vi "CANOpen_NMT_Write HW Outputs.vi"(8 "error in":errorcluster, 9 "Node Ids":T1, 10 "Hardware Output FIFO":refnum<k33>, 11 "Channel Pairs":T2 {"Chan Refs"."Data Reference" format="%.0x"}) -> (0 "error out":errorcluster, 2 "Write Occured":bool, 3 "Channel Pairs":T2 {"Chan Refs"."Data Reference" format="%.0x"})   [LabVIEW 2021, in "CANOpen Addon Engine.lvlib"]
uses:
  CANOpen Addon Engine.lvlib
  CanOpen_NMT_HWOut_ChannelPairs.ctl
  <vilib>/NI VeriStand/Custom Device API/Block Data Reference.ctl
  <vilib>/NI VeriStand/Custom Device API/Data Reference.ctl
  CanOpen_Main Node Ids.ctl
  <vilib>/NI VeriStand/Custom Device API/Global Data Refs.vi
  <vilib>/NI VeriStand/Custom Device API/Custom Device API.lvlib
  Debug/SubVIs/Global debug.vi
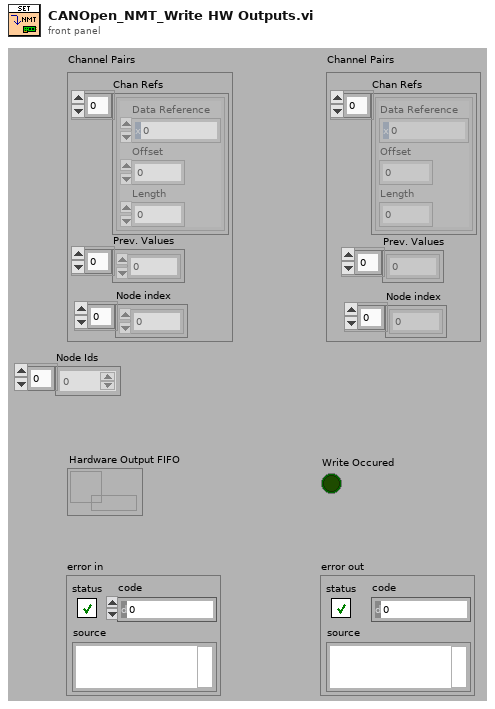
[diagram p1: front panel]
types:
  T1 = typedef "CANOpen Addon Engine.lvlib/CanOpen_Main Node Ids.ctl" = u8[]
  T2 = typedef "CANOpen Addon Engine.lvlib/CanOpen_NMT_HWOut_ChannelPairs.ctl" = cluster{"Chan Refs":T3[], "Prev. Values":dbl[], "Node index":dbl[]}
  T3 = typedef "Custom Device API.lvlib/Block Data Reference.ctl" = cluster{"Data Reference":T4, "Offset":u64, "Length":u64}
  T4 = typedef "Custom Device API.lvlib/Data Reference.ctl" = i32
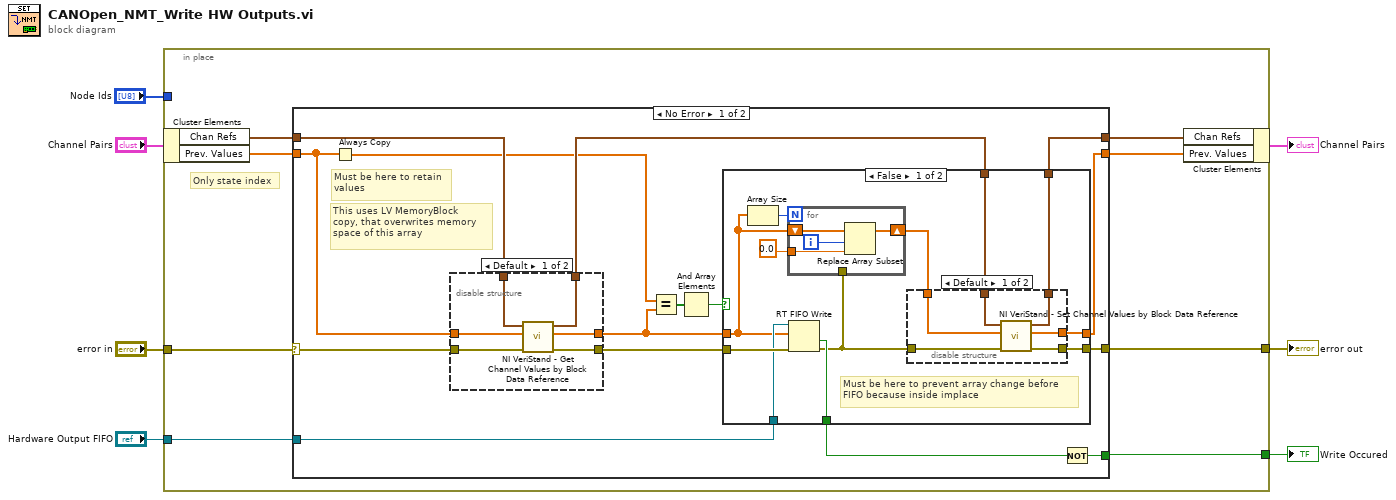
[diagram p0: block diagram]
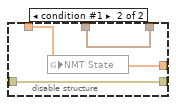
[diagram p2: hidden frame]
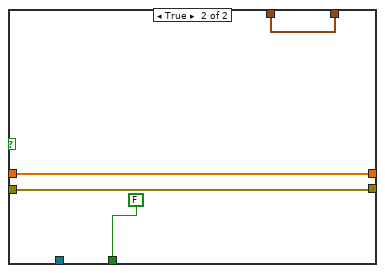
[diagram p3: hidden frame]
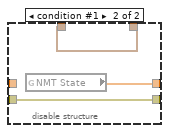
[diagram p4: hidden frame]
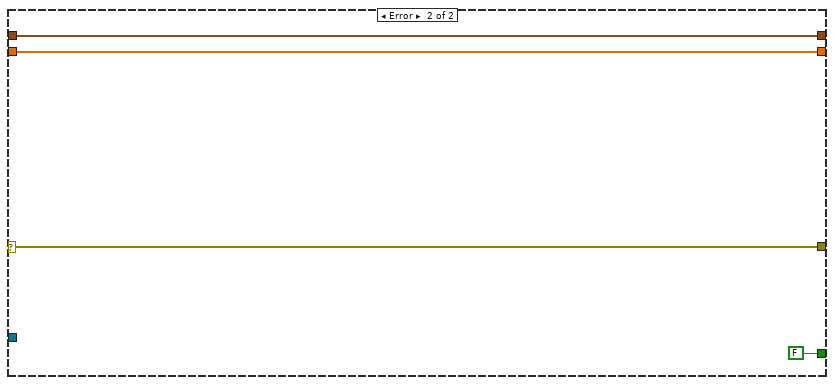
[diagram p5: hidden frame]
diagram:
  n1 = in-place {
    in-place-border: [w15] -> w7
    in-place-border: [w14] -> w6
    in-place-border: "error in" -> [w11]
    in-place-border: "Hardware Output FIFO" -> [w8]
    in-place-border: "Node Ids" -> [_]
    # "Only state index"
    n2 = in-place-cluster #1("Channel Pairs") -> ("Chan Refs"=w13:T3[], "Prev. Values"=w10:dbl[])
    n3 = case shown="No Error" w11 {
      selector: w11 -> [w27 w72]
      tunnel: [w28 w72] -> w15
      tunnel: [w19 w69] -> w9
      tunnel: [w29 FALSE ("C Read Occured?")] -> w14
      tunnel: w13 -> [w25 w70]
      tunnel: [w20 w70] -> w12
      tunnel: w10 -> [w16 w69]
      tunnel: w8 -> [w24 _]
      frame No Error {
        # "This uses LV MemoryBlock\ncopy, that overwrites memory\nspace of this array"
        # "Must be here to retain\nvalues"
        n4 = Always Copy(1:w16) -> (0:w17:dbl[])
        n5 = disable-structure shown="Default" {
          disable-tunnel: w27 -> [w65 w68]
          disable-tunnel: [w61 w68] -> w26
          disable-tunnel: w25 -> [w64 w67]
          disable-tunnel: [w63 w67] -> w21
          disable-tunnel: w16 -> [w62 _]
          disable-tunnel: [w60 w66] -> w18
          frame condition #0 (active) {
            n6 = call <vilib>:"NI VeriStand - Get Channel Values by Block Data Reference.vi"("error in (no error)"=w65, "Values Array in"=w62, "Block Data Ref"=w64) -> ("error out"=w61:errorcluster, "Values Array out"=w60:dbl[], "Block Data Ref dup"=w63:T3[])  [unwired: 6 in]
          }
          frame condition #1 {
            n7 = global read "Global debug.vi" "NMT State"() -> (w66:dbl[])
          }
        }
        n8 = Equal?(x=w17, y=w18) -> (x = y?=w23:bool[])
        n9 = And Array Elements(Boolean array=w23) -> (logical AND=w22:bool)
        n10 = case shown="False" w22 {
          tunnel: [w37 FALSE ("timed out?")] -> w30
          tunnel: [w40 w58] -> w28
          tunnel: w26 -> [w42 w58]
          tunnel: w24 -> [w41 _]
          tunnel: w18 -> [w32 w56]
          tunnel: w21 -> [w39 w57]
          tunnel: [w38 w57] -> w20
          tunnel: [w36 w56] -> w19
          frame False {
            # "Must be here to prevent array change before\nFIFO because inside implace"
            n11 = Array Size(array=w32) -> (size(s)=w31:i32)
            n12 = RT FIFO Write(0:w41, 1:w32, 3:w42) -> (10:w37:bool, 11:w35:errorcluster)  [unwired: 2 in, 2 out]
            n13 = for {
              N: w31 -> [_]
              tunnel: w35 -> [_]
              tunnel: 0.0 ("Channel Data Reference") -> [w44]
              shift-right: [w43] -> w33
              shift-left: w32 -> [w46]
              i -> [w45]
              n14 = Replace Array Subset(array=w46, new element=w44, index=w45) -> (w43:dbl[])
            }
            n15 = disable-structure shown="Default" {
              disable-tunnel: w35 -> [w52 w54]
              disable-tunnel: [w51 w54] -> w40
              disable-tunnel: w39 -> [w50 w55]
              disable-tunnel: [w49 w55] -> w38
              disable-tunnel: w33 -> [w48 w53]
              disable-tunnel: [w47 w53] -> w36
              frame condition #0 (active) {
                n16 = call <vilib>:"NI VeriStand - Set Channel Values by Block Data Reference.vi"("error in (no error)"=w52, "Values Array in"=w48, "Block Data Ref"=w50) -> ("error out"=w51:errorcluster, "Values Array out"=w47:dbl[], "Block Data Ref dup"=w49:T3[])  [unwired: 6 in]
              }
              frame condition #1 {
                n17 = global write "Global debug.vi" "NMT State"(w53) -> ()
              }
            }
          }
          frame True {
          }
        }
        n18 = Not(x=w30) -> (.not. x?=w29:bool)
      }
      frame Error {
      }
    }
    n19 = in-place-cluster #1("Chan Refs"=w12, "Prev. Values"=w9) -> (→"Channel Pairs":T2)
  }
  "error out" <- w7
  "Write Occured" <- w6
